vi "Init.vi"(8 "error in (no error)":errorcluster, 11 "File Path":path) -> (0 "error out":errorcluster)   [LabVIEW 2018, in "Receipt Parsing.lvlib"]
uses:
  Receipt Parsing.lvlib
  Action.ctl
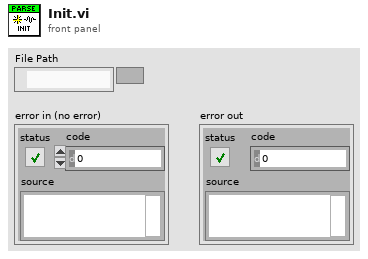
[diagram p1: front panel]
types:
  T1 = typedef "Receipt Parsing.lvlib/Action.ctl" = enum16{"Init", "Read Image Text", "Close"}
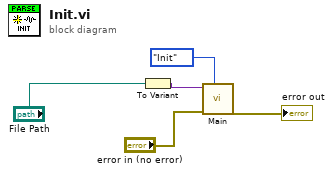
[diagram p0: block diagram]
diagram:
  n1 = To Variant(anything="File Path") -> (Variant=w3:variant)
  n2 = call "Main.vi"("Action"=Action."Init", "Error In"="error in (no error)", "Data In"=w3) -> ("Error Out"=→"error out":errorcluster)  [unwired: 7 in, 1 out]
